vi "Slider Position Chasing Top Min.vi"(5 "Asigned Slider":i32=1, 7 "Chasing Active Slider":bool=TRUE, 8 "Position Compensate":cluster{"Array 2":dbl[]}[](array[cluster]) {"Array 2" format="%#_f"}, 10 "Chasing Group":cluster{"Array 2":refnum<vi>[]}[](array[cluster]), 11 "Slide Reference In":refnum<vi>) -> (3 "Slide Reference Out":refnum<vi>)   [LabVIEW 2024]
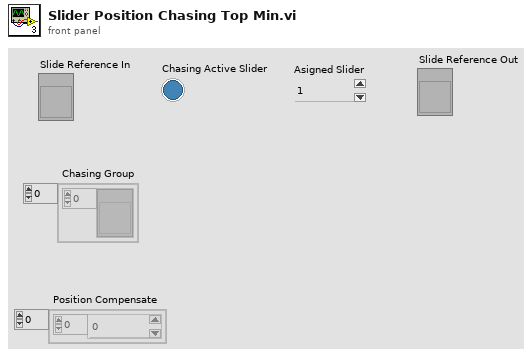
[diagram p1: front panel]
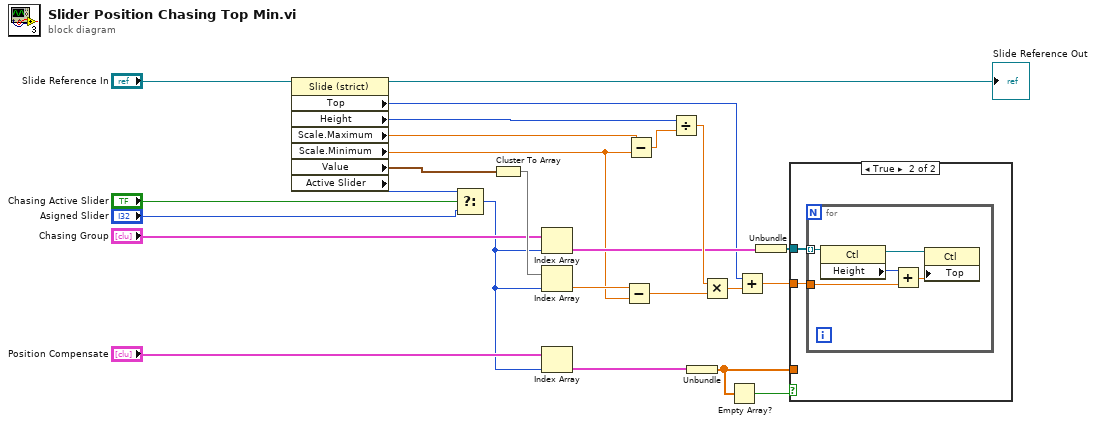
[diagram p0: block diagram]
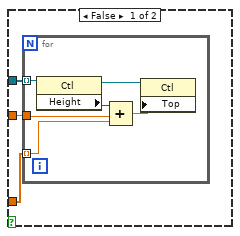
[diagram p2: hidden frame]
diagram:
  n1 = property class="Slide (strict)"(reference="Slide Reference In") -> (reference out=→"Slide Reference Out":refnum<vi>, "Top"=w4:i32, "Height"=w24:u32, "Scale.Maximum"=w23:dbl, "Scale.Minimum"=w2:dbl, "Value"=w18:cluster{dbl, dbl, dbl}, "Active Slider"=w7:i32)  [unwired: 1 in, 1 out]
  n2 = Select(t=w7, s="Chasing Active Slider", f="Asigned Slider") -> (s? t:f=w6:i32)
  n3 = Cluster To Array(cluster=w18) -> (array=w17:dbl[])
  n4 = Index Array(array="Chasing Group", index=w6) -> (element=w15:cluster{"Array 2":refnum<vi>[]})
  n5 = Index Array(array=w17, index=w6) -> (element=w3:dbl)
  n6 = Index Array(array="Position Compensate", index=w6) -> (element=w12:cluster{"Array 2":dbl[]})
  n7 = Subtract(x=w3, y=w2) -> (x-y=w1:dbl)
  n8 = Subtract(x=w23, y=w2) -> (x-y=w25:dbl)
  n9 = Divide(x=w24, y=w25) -> (x/y=w21:dbl)
  n10 = Unbundle(w12) -> ("Array 2"=w10:dbl[])
  n11 = Multiply(x=w21, y=w1) -> (x*y=w22:dbl)
  n12 = Empty Array?(array=w10) -> (empty?=w11:bool)
  n13 = Add(x=w4, y=w22) -> (x+y=w20:dbl)
  n14 = Unbundle(w15) -> ("Array 2"=w14:refnum<vi>[])
  n15 = case shown="True" w11 {
    tunnel: w20 -> [w28 w35]
    tunnel: w14 -> [w27 w36]
    tunnel: w10 -> [w26 _]
    frame False {
      n16 = for {
        tunnel: w28 -> [w30]
        tunnel: w27 -> [w31] mode=indexing
        tunnel: w26 -> [w29] mode=indexing
        n17 = property class="Ctl"(reference=w31) -> (reference out=w33:refnum<vi>, "Height"=w32:u32)  [unwired: 1 in, 1 out]
        n18 = Compound Arithmetic op=ADD(w32, w30, w29) -> (w34:dbl)
        n19 = property class="Ctl"(reference=w33, "Top"=w34) -> ()  [unwired: 1 in, 2 out]
      }
    }
    frame True {
      n20 = for {
        tunnel: w35 -> [w39]
        tunnel: w36 -> [w40] mode=indexing
        n21 = property class="Ctl"(reference=w40) -> (reference out=w41:refnum<vi>, "Height"=w38:u32)  [unwired: 1 in, 1 out]
        n22 = Add(x=w38, y=w39) -> (x+y=w37:dbl)
        n23 = property class="Ctl"(reference=w41, "Top"=w37) -> ()  [unwired: 1 in, 2 out]
      }
    }
  }
